vi "Init IMU.vi"(9 "# UART Butes":dbl, 10 "Num Data Points \nto train PCA":i32=5000) -> (2 "VISA resource name out":refnum<visa-resource-name>)   [LabVIEW 2018]
uses:
  <vilib>/myRIO/Instrument Drivers/Onboard IO/UART/typedef/VISA Configuration.ctl
  <vilib>/Instr/_visa.llb/VISA Flush IO Buffer Mask.ctl
  <vilib>/Instr/_visa.llb/VISA Configure Serial Port (Instr).vi
  <vilib>/myRIO/Instrument Drivers/Onboard IO/UART/UART.lvlib
panel:
  out "Training PCA":bool
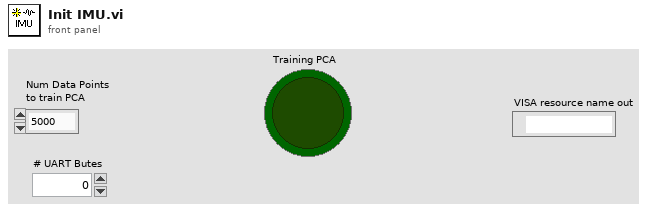
[diagram p1: front panel]
types:
  T1 = typedef "UART.lvlib/VISA Configuration.ctl" = cluster{"baud rate (9600)":u32, "data bits (8)":u16, "parity (0:none)":enum16{"None", "Odd", "Even", "Mark", "Space"}, "stop bits (10: 1 bit)":u16, "flow control (0:none)":u16, "termination char\n(0xA = '\\n' = LF) ":u8, "Enable Termination\nChar (T)":bool, "timeout (10sec)":u32}
  T2 = typedef "VISA Flush IO Buffer Mask.ctl" = u16
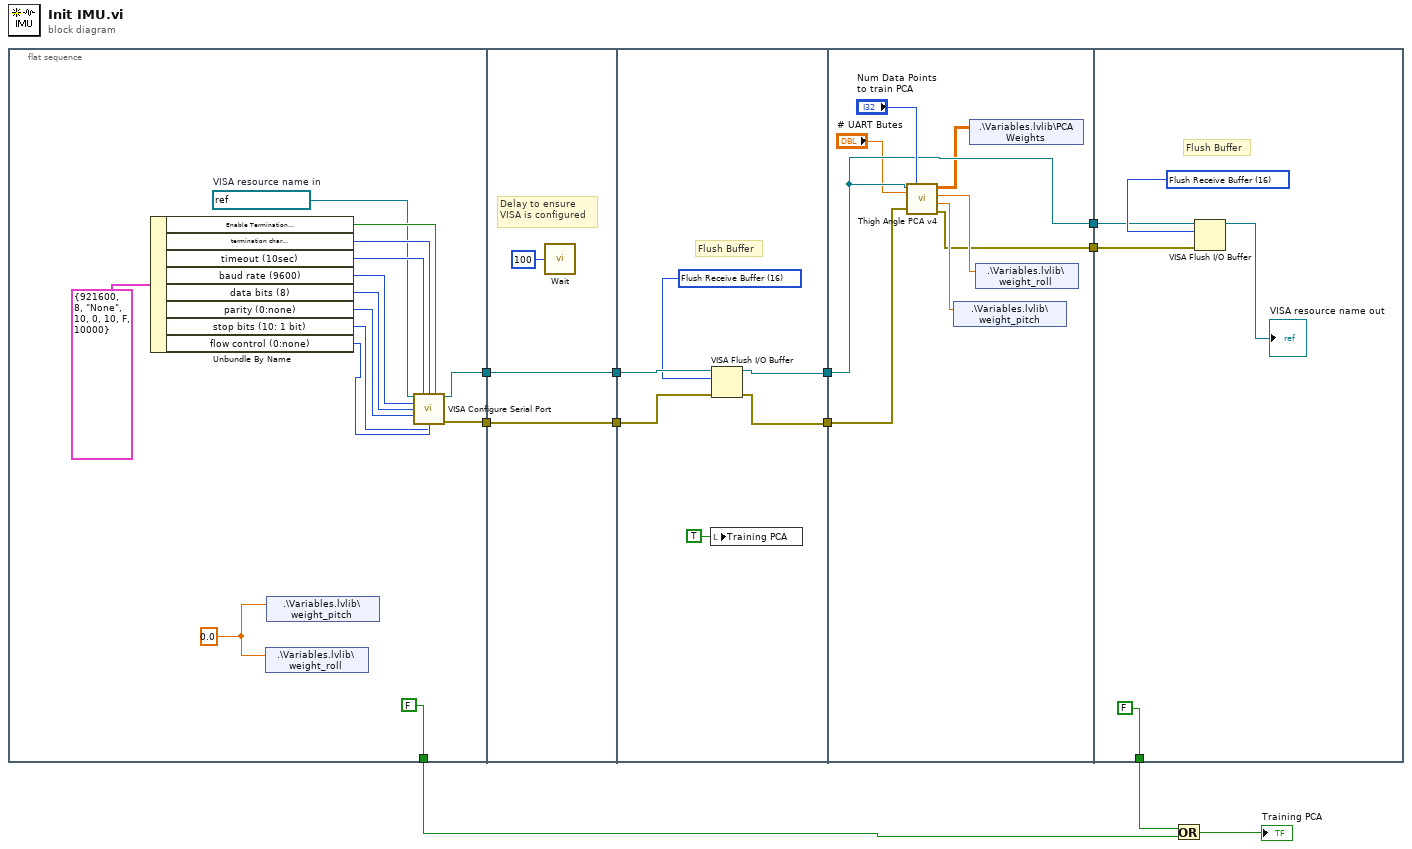
[diagram p0: block diagram]
diagram:
  n1 = flat-sequence {
    tunnel: [w14] -> w11
    tunnel: [w15] -> w10
    tunnel: [FALSE] -> w3
    tunnel: w11 -> [w26]
    tunnel: [w26] -> w9
    tunnel: w10 -> [w28]
    tunnel: [w28] -> w8
    tunnel: w9 -> [w32]
    tunnel: [w31] -> w7
    tunnel: w8 -> [w34]
    tunnel: [w33] -> w6
    tunnel: w7 -> [w39]
    tunnel: w6 -> [w41]
    tunnel: [w36] -> w5
    tunnel: [w41] -> w4
    tunnel: w5 -> [w45]
    tunnel: w4 -> [w44]
    tunnel: [FALSE] -> w2
    frame #0 {
      w13 = 0.0 ("weight_pitch")
      w16 = refnum<visa-resource-name> "ASRL2::INSTR"  # VISA resource name in
      n2 = Unbundle By Name(T1 {"baud rate (9600)"=921600, "data bits (8)"=8, "parity (0:none)"=enum."None", "stop bits (10: 1 bit)"=10, "flow control (0:none)"=0, "termination char\n(0xA = '\\n' = LF) "=10, "Enable Termination\nChar (T)"=FALSE, "timeout (10sec)"=10000} ("VISA Configuration")) -> ("Enable Termination\nChar (T)"=w22:bool, "termination char\n(0xA = '\\n' = LF)"=w23:u8, "timeout (10sec)"=w17:u32, "baud rate (9600)"=w20:u32, "data bits (8)"=w19:u16, "parity (0:none)"=w18:enum16{"None", "Odd", "Even", "Mark", "Space"}, "stop bits (10: 1 bit)"=w24:u16, "flow control (0:none)"=w25:u16)
      n3 = shared-variable ".\\Variables.lvlib\\weight_roll"(w13) -> ()  [unwired: 1 in, 1 out]
      n4 = shared-variable ".\\Variables.lvlib\\weight_pitch"(w13) -> ()  [unwired: 1 in, 1 out]
      n5 = call-poly "VISA Configure Serial Port"("VISA resource name"=w16, "timeout (10sec)"=w17, "termination char\n(0xA = '\\n' = LF)"=w23, "Enable Termination\nChar (T)"=w22, "baud rate (9600)"=w20, "data bits (8)"=w19, "parity (0:none)"=w18, "stop bits (10: 1 bit)"=w24, "flow control (0:none)"=w25) -> ("VISA resource name out"=w15:refnum<visa-resource-name>, "error out"=w14:errorcluster)  [unwired: 5 in]
    }
    frame #1 {
      # "Delay to ensure\nVISA is configured"
      n6 = call "Wait"("Count(mSec)"=u32 100) -> ()  [unwired: 1 out]
    }
    frame #2 {
      w30 = T2 16 items=["Flush Receive Buffer"=16, "Write Transmit Buffer to Device"=32, "Flush Receive Buffer (No I/O)"=64, "Flush Transmit Buffer"=128] ("Mask")
      # "Flush Buffer"
      n7 = local write "Training PCA"(TRUE ("Training PCA")) -> ()
      n8 = VISA Flush I/O Buffer(VISA resource name=w34, mask (16)=w30, error in (no error)=w32) -> (VISA resource name out=w33:refnum<visa-resource-name>, error out=w31:errorcluster)
    }
    frame #3 {
      n9 = call "Thigh Angle PCA v4.vi"("Num Data Point"="Num Data Points \nto train PCA", "error in (no error)"=w39, "byte count"="# UART Butes", "VISA resource name"=w41) -> ("error out"=w36:errorcluster, "w_pitch"=w38:dbl, "w_roll"=w37:dbl, "weights"=w35:dbl[][])  [unwired: 4 in]
      n10 = shared-variable ".\\Variables.lvlib\\weight_pitch"(w38) -> ()  [unwired: 1 in, 1 out]
      n11 = shared-variable ".\\Variables.lvlib\\PCA Weights"(w35) -> ()  [unwired: 1 in, 1 out]
      n12 = shared-variable ".\\Variables.lvlib\\weight_roll"(w37) -> ()  [unwired: 1 in, 1 out]
    }
    frame #4 {
      w47 = T2 16 items=["Flush Receive Buffer"=16, "Write Transmit Buffer to Device"=32, "Flush Receive Buffer (No I/O)"=64, "Flush Transmit Buffer"=128] ("Mask")
      # "Flush Buffer"
      n13 = VISA Flush I/O Buffer(VISA resource name=w44, mask (16)=w47, error in (no error)=w45) -> (VISA resource name out=→"VISA resource name out":refnum<visa-resource-name>)  [unwired: 1 out]
    }
  }
  n14 = Or(x=w2, y=w3) -> (x .or. y?=→"Training PCA":bool)
